vi "write to RF synth bd.vi"(0 "Address Byte":u8, 1 "BD 2 Byte":u8, 2 "BD 1 Byte":u8) -> ()   [LabVIEW 2013]
uses:
  <vilib>/rvi/eio/common/nirviEmuTemplateMethod_errors.vi
  <vilib>/eio/EIONode/EIONode.xnode
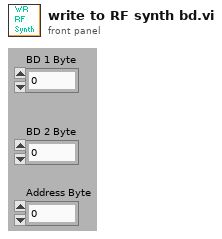
[diagram p1: front panel]
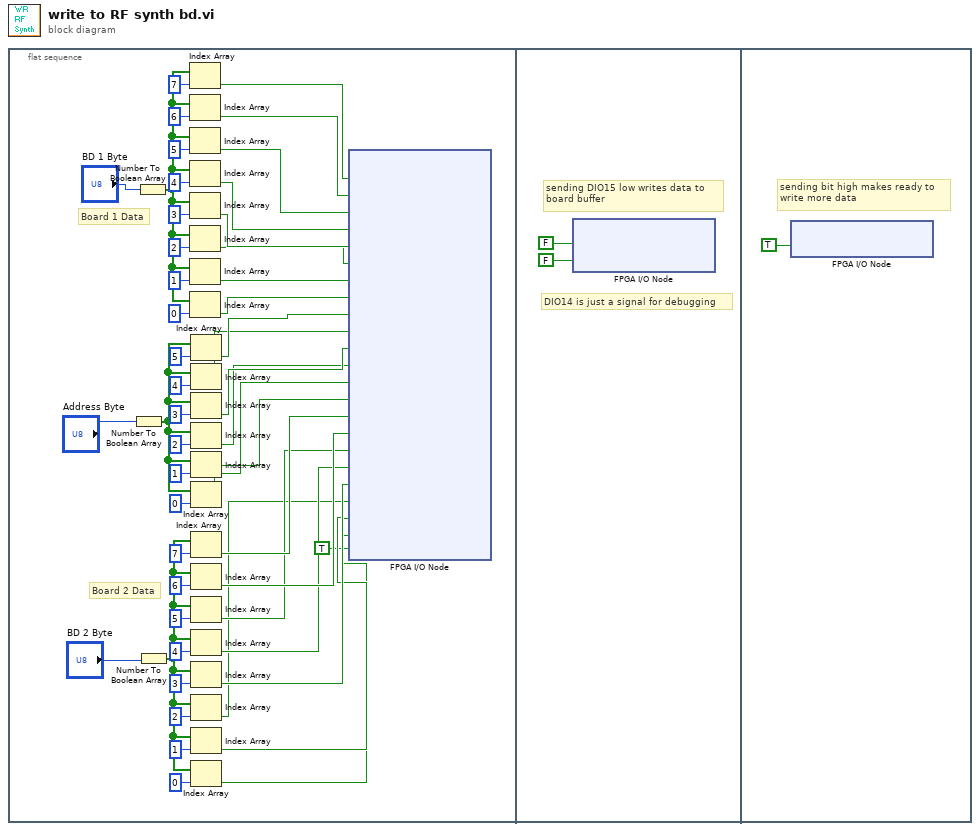
[diagram p0: block diagram]
diagram:
  n1 = flat-sequence {
    frame #0 {
      # "Board 1 Data"
      # "Board 2 Data"
      n2 = Number To Boolean Array(number="Address Byte") -> (Boolean array=w50:bool[])
      n3 = Number To Boolean Array(number="BD 1 Byte") -> (Boolean array=w51:bool[])
      n4 = Number To Boolean Array(number="BD 2 Byte") -> (Boolean array=w21:bool[])
      n5 = Index Array(array=w51, index=7) -> (element=w35:bool)
      n6 = Index Array(array=w51, index=6) -> (element=w34:bool)
      n7 = Index Array(array=w51, index=5) -> (element=w33:bool)
      n8 = Index Array(array=w51, index=4) -> (element=w32:bool)
      n9 = Index Array(array=w51, index=3) -> (element=w31:bool)
      n10 = Index Array(array=w51, index=2) -> (element=w30:bool)
      n11 = Index Array(array=w51, index=1) -> (element=w29:bool)
      n12 = Index Array(array=w51, index=0) -> (element=w28:bool)
      n13 = Index Array(array=w50, index=5) -> (element=w27:bool)
      n14 = Index Array(array=w50, index=4) -> (element=w26:bool)
      n15 = Index Array(array=w50, index=3) -> (element=w25:bool)
      n16 = Index Array(array=w50, index=2) -> (element=w24:bool)
      n17 = Index Array(array=w50, index=1) -> (element=w23:bool)
      n18 = Index Array(array=w50, index=0) -> (element=w22:bool)
      n19 = Index Array(array=w21, index=7) -> (element=w12:bool)
      n20 = Index Array(array=w21, index=6) -> (element=w11:bool)
      n21 = Index Array(array=w21, index=5) -> (element=w10:bool)
      n22 = Index Array(array=w21, index=4) -> (element=w9:bool)
      n23 = Index Array(array=w21, index=3) -> (element=w8:bool)
      n24 = Index Array(array=w21, index=2) -> (element=w7:bool)
      n25 = Index Array(array=w21, index=1) -> (element=w6:bool)
      n26 = Index Array(array=w21, index=0) -> (element=w5:bool)
      n27 = xnode "FPGA I/O Node"("Connector1/DIO0"=w35, "Connector1/DIO1"=w34, "Connector1/DIO2"=w33, "Connector1/DIO3"=w32, "Connector1/DIO4"=w31, "Connector1/DIO5"=w30, "Connector1/DIO6"=w29, "Connector1/DIO7"=w28, "Connector1/DIO8"=w27, "Connector1/DIO9"=w26, "Connector1/DIO10"=w25, "Connector1/DIO11"=w24, "Connector1/DIO12"=w23, "Connector1/DIO13"=w22, "Connector1/DIO20"=w12, "Connector1/DIO21"=w11, "Connector1/DIO22"=w10, "Connector1/DIO23"=w9, "Connector1/DIO24"=w8, "Connector1/DIO25"=w7, "Connector1/DIO26"=w6, "Connector1/DIO27"=w5, "Connector1/DIO14"=TRUE) -> ()  [unwired: 23 in, 23 out]
    }
    frame #1 {
      # "DIO14 is just a signal for debugging"
      # "sending DIO15 low writes data to \nboard buffer"
      n28 = xnode "FPGA I/O Node"("Connector1/DIO15"=FALSE, "Connector1/DIO14"=FALSE) -> ()  [unwired: 2 in, 2 out]
    }
    frame #2 {
      # "sending bit high makes ready to\nwrite more data"
      n29 = xnode "FPGA I/O Node"("Connector1/DIO15"=TRUE) -> ()  [unwired: 1 in, 1 out]
    }
  }
